vi "IsAimingGoal.vi"(0 "object in":refnum<class "DefendGoalTactic.lvclass">, 2 "Game":refnum<class "Game.lvclass">, 4 "Robot position":dbl[](array[numeric]), 5 "error in (no error)":errorcluster) -> (14 "object out":refnum<class "DefendGoalTactic.lvclass">, 16 "IsAiming":bool, 18 "Y aiming in goal coerced":dbl, 19 "error out":errorcluster)   [LabVIEW 2024, in "DefendGoalTactic.lvclass"]
uses:
  DefendGoalTactic.lvclass
  Game_class/Game.lvclass
  Game_class/Game.lvclass/Game.ctl
  Object_class/Object.lvclass/Object.ctl
  Field_class/Field.lvclass/Field.ctl
  Object_class/Read y.vi
  Object_class/Read x.vi
  Object_class/Read position(x,y).vi
  Field_class/Read ourGoalPosition.vi
  Game_class/Read BallRef.vi
  Game_class/Read FieldRef.vi
  Ball_class/Ball.lvclass
  C:/Users/ROBOIME2/Documents/SSL ROBOIME/SSL_AI/Object_class/Object.lvclass
  Field_class/Field.lvclass
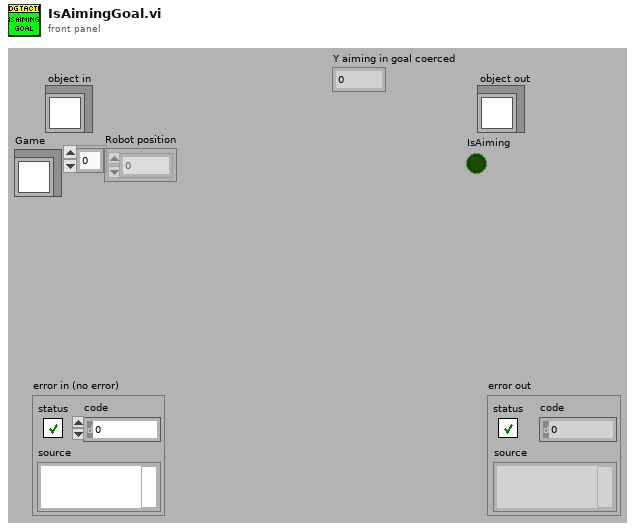
[diagram p1: front panel]
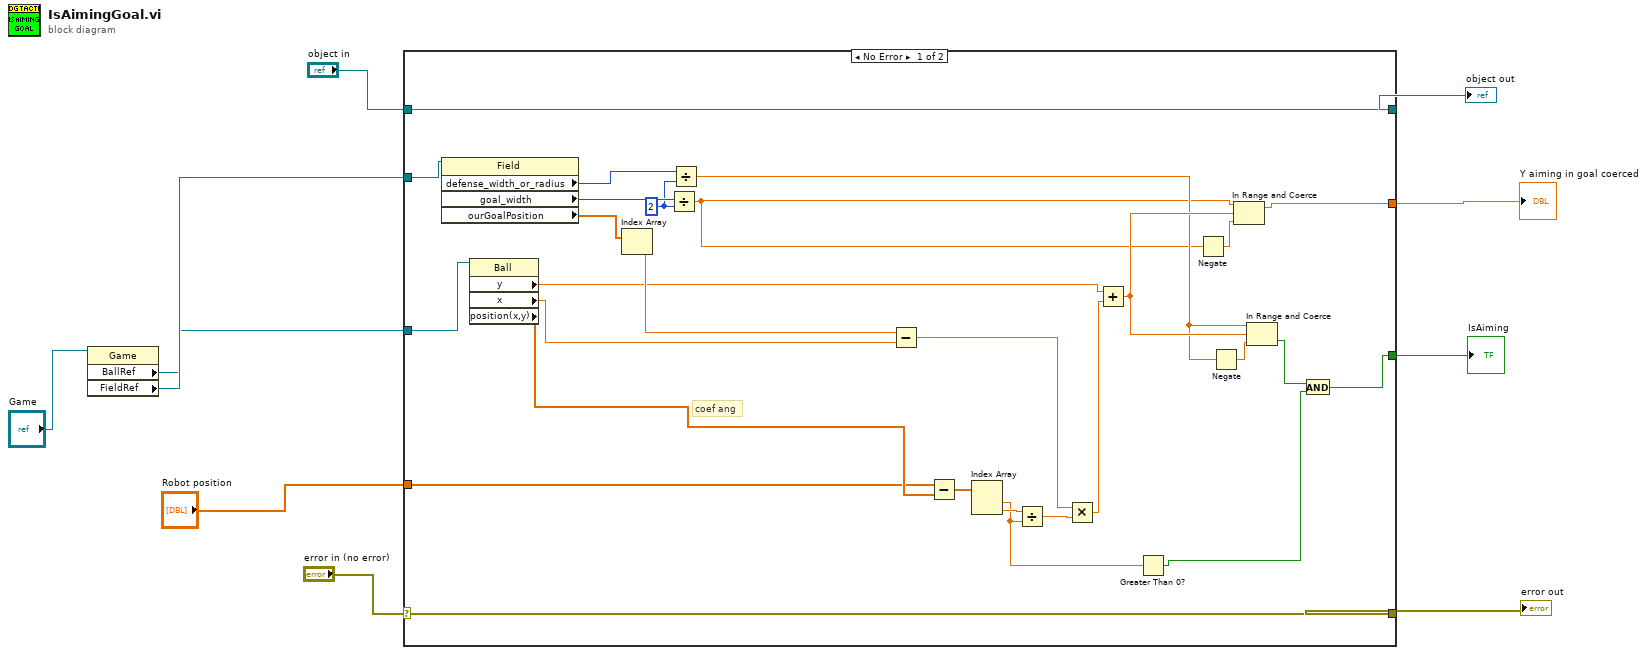
[diagram p0: block diagram]
diagram:
  n1 = property class="Game"(reference="Game") -> ("BallRef"=w3:refnum<class "Ball.lvclass">, "FieldRef"=w4:refnum<class "Field.lvclass">)  [unwired: 1 in, 2 out]
  n2 = case shown="No Error" "error in (no error)" {
    selector: "error in (no error)" -> [w37 w40]
    tunnel: [w37 w40] -> w8
    tunnel: [w38 w39] -> w7
    tunnel: "object in" -> [w38 w39]
    tunnel: [w11 _] -> w10
    tunnel: w4 -> [w24 _]
    tunnel: w3 -> [w23 _]
    tunnel: "Robot position" -> [w22 _]
    tunnel: [w19 _] -> w1
    frame No Error {
      w21 = 2 ("y")
      # "coef ang"
      n3 = property class="Field"(reference=w24) -> ("defense_width_or_radius"=w20:i32, "goal_width"=w34:i32, "ourGoalPosition"=w36:dbl[])  [unwired: 1 in, 2 out]
      n4 = property class="Ball"(reference=w23) -> ("y"=w26:dbl, "x"=w28:dbl, "position(x,y)"=w32:dbl[])  [unwired: 1 in, 2 out]
      n5 = Index Array(array=w36) -> (element=w35:dbl)  [unwired: 1 in]
      n6 = Divide(x=w34, y=w21) -> (x/y=w15:dbl)
      n7 = Divide(x=w20, y=w21) -> (x/y=w17:dbl)
      n8 = Subtract(x=w35, y=w28) -> (x-y=w27:dbl)
      n9 = Subtract(x=w22, y=w32) -> (x-y=w31:dbl[])
      n10 = Index Array(array=w31) -> (element #1=w14:dbl, element #2=w30:dbl)  [unwired: 2 in]
      n11 = Divide(x=w30, y=w14) -> (x/y=w29:dbl)
      n12 = Multiply(x=w27, y=w29) -> (x*y=w25:dbl)
      n13 = Add(x=w26, y=w25) -> (x+y=w18:dbl)
      n14 = Greater Than 0?(x=w14) -> (x > 0?=w12:bool)
      n15 = Negate(x=w15) -> (-x=w16:dbl)
      n16 = Negate(x=w17) -> (-x=w33:dbl)
      n17 = In Range and Coerce(upper limit=w15, x=w18, lower limit=w16) -> (coerced(x)=w19:dbl)  [unwired: 1 out]
      n18 = In Range and Coerce(upper limit=w17, x=w18, lower limit=w33) -> (In Range?=w13:bool)  [unwired: 1 out]
      n19 = And(x=w13, y=w12) -> (x .and. y?=w11:bool)
    }
    frame Error {
    }
  }
  "error out" <- w8
  "object out" <- w7
  "IsAiming" <- w10
  "Y aiming in goal coerced" <- w1
